vi "test SSL Client HTTPS Request to Google.vi"(8 "error in (no error)":errorcluster, 11 "TestCase in":refnum<class "test SSL Client.lvclass">) -> (0 "error out":errorcluster, 3 "TestCase out":refnum<class "test SSL Client.lvclass">)   [LabVIEW 2013, in "test SSL Client.lvclass"]
uses:
  test SSL Client.lvclass
  <vilib>/addons/_JKI Toolkits/VI Tester/TestCase.llb/TestCase.lvclass
  SSL_Lib/BIO/BIO.lvclass
  <vilib>/Wiresmith Technology/VITAC (VI Tester Advanced Comparisons)/VITAC.lvlib
  SSL_Lib/SSL-Context/SSL-Context.lvclass
  SSL_Lib/SSL/SSL.lvclass
  SSL_Lib/SSL/SSL_Mode.ctl
  suite SSL Client/suite SSL Client/SSL Context.vi
  suite SSL Client/suite SSL Client/suite SSL Client.lvclass
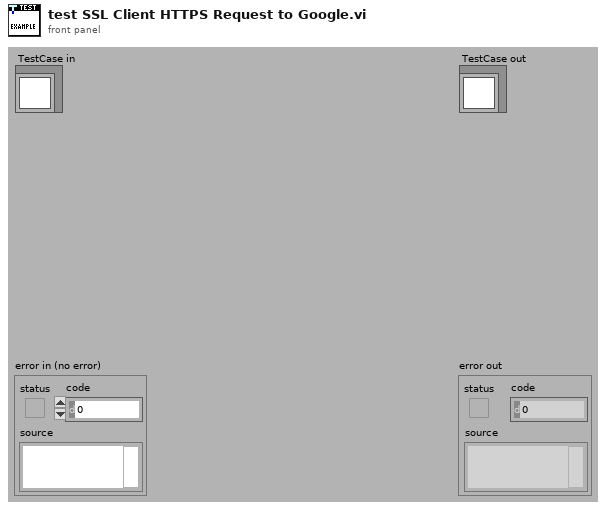
[diagram p1: front panel]
types:
  T1 = typedef "SSL_Lib.lvlib/SSL.lvclass/SSL_Mode.ctl" = i32
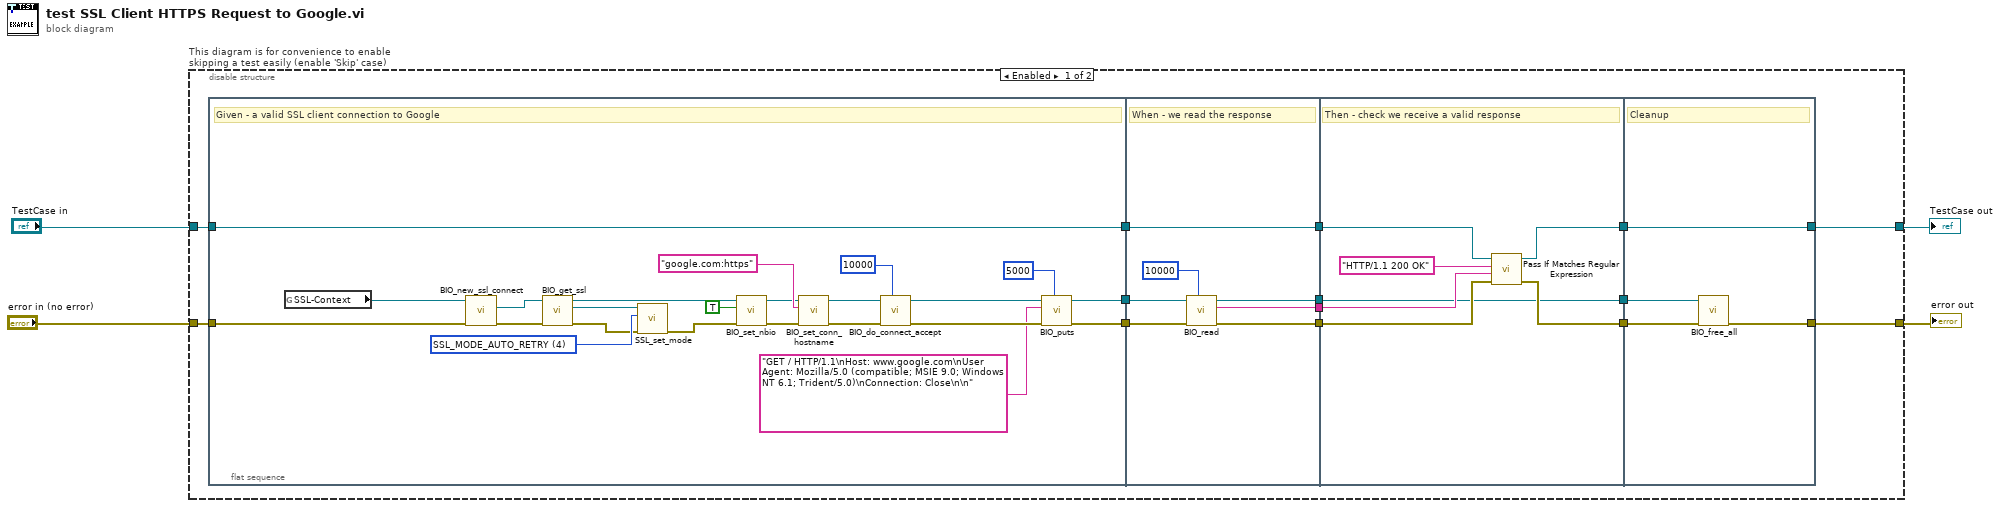
[diagram p0: block diagram]
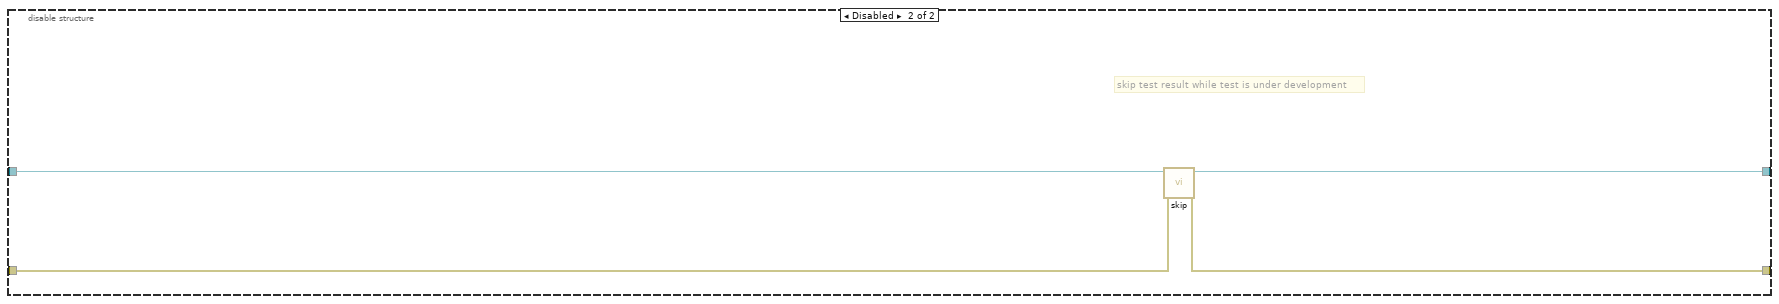
[diagram p2: hidden frame]
diagram:
  n1 = disable-structure "This diagram is for convenience to enable skipping a test easily (enable 'Skip' case)" shown="Enabled" {
    disable-tunnel: "TestCase in" -> [w12 w63]
    disable-tunnel: [w11 w61] -> w1
    disable-tunnel: [w10 w62] -> w3
    disable-tunnel: "error in (no error)" -> [w13 w60]
    frame Enabled {
      n2 = flat-sequence {
        tunnel: w13 -> [w27]
        tunnel: w12 -> [w36]
        tunnel: [w36] -> w18
        tunnel: [w35] -> w9
        tunnel: [w34] -> w8
        tunnel: [w48] -> w17
        tunnel: [w45] -> w16
        tunnel: w18 -> [w48]
        tunnel: w9 -> [w47]
        tunnel: w8 -> [w46]
        tunnel: [w44] -> w7
        tunnel: [w43] -> w6
        tunnel: [w53] -> w15
        tunnel: [w52] -> w14
        tunnel: w17 -> [w54]
        tunnel: w16 -> [w55]
        tunnel: w7 -> [w51]
        tunnel: w6 -> [w49]
        tunnel: [w49] -> w5
        tunnel: [w57] -> w10
        tunnel: [w59] -> w11
        tunnel: w15 -> [w59]
        tunnel: w14 -> [w58]
        tunnel: w5 -> [w56]
        frame #0 {
          w29 = T1 4 items=["None"=0, "SSL_MODE_ENABLE_PARTIAL_WRITE"=1, "SSL_MODE_ACCEPT_MOVING_WRITE_BUFFER"=2, "SSL_MODE_AUTO_RETRY"=4, "SSL_MODE_RELEASE_BUFFERS"=16, "SSL_MODE_SEND_FALLBACK_SCSV"=128] ("Mode")
          # "Given - a valid SSL client connection to Google"
          n3 = global read "SSL Context.vi" "SSL-Context"() -> (w26:refnum<class "SSL-Context.lvclass">)
          n4 = call "BIO_new_ssl_connect.vi"("error in (no error)"=w27, "SSL-Context in"=w26) -> ("error out"=w31:errorcluster, "BIO out"=w32:refnum<class "BIO.lvclass">)  [unwired: 7 in, 1 out]
          n5 = call "BIO_get_ssl.vi"("error in (no error)"=w31, "BIO in"=w32) -> ("error out"=w28:errorcluster, "SSL out"=w30:refnum<class "SSL.lvclass">, "BIO out"=w21:refnum<class "BIO.lvclass">)  [unwired: 7 in]
          n6 = call "SSL_set_mode.vi"("error in (no error)"=w28, "Mode"=w29, "SSL in"=w30) -> ("error out"=w24:errorcluster)  [unwired: 7 in, 1 out]
          n7 = call "BIO_set_nbio.vi"("error in (no error)"=w24, "Non-Blocking?"=TRUE, "BIO in"=w21) -> ("error out"=w22:errorcluster, "BIO out"=w23:refnum<class "BIO.lvclass">)  [unwired: 7 in]
          n8 = call "BIO_set_conn_hostname.vi"("error in (no error)"=w22, "Hostname"="google.com:https", "BIO in"=w23) -> ("error out"=w40:errorcluster, "BIO out"=w33:refnum<class "BIO.lvclass">)  [unwired: 7 in]
          n9 = call "BIO_do_connect_accept.vi"("Timeout (10000ms)"=u32 10000, "error in (no error)"=w40, "BIO in"=w33) -> ("error out"=w38:errorcluster, "BIO out"=w37:refnum<class "BIO.lvclass">)  [unwired: 7 in]
          n10 = call "BIO_puts.vi"("Timeout (10000ms)"=u32 5000, "error in (no error)"=w38, "String to write"="GET / HTTP/1.1\nHost: www.google.com\nUser Agent: Mozilla/5.0 (compatible; MSIE 9.0; Windows NT 6.1; Trident/5.0)\nConnection: Close\n\n", "BIO in"=w37) -> ("error out"=w35:errorcluster, "BIO out"=w34:refnum<class "BIO.lvclass">)  [unwired: 6 in]
        }
        frame #1 {
          # "When - we read the response"
          n11 = call "BIO_read.vi"("Timeout (10000ms)"=u32 10000, "error in (no error)"=w47, "BIO in"=w46) -> ("error out"=w45:errorcluster, "String read"=w44:string, "BIO out"=w43:refnum<class "BIO.lvclass">)  [unwired: 6 in]
        }
        frame #2 {
          # "Then - check we receive a valid response"
          n12 = call <vilib>:"Pass If Matches Regular Expression.vi"("error in (no error)"=w55, "actual"=w51, "regular expression"="HTTP/1.1 200 OK", "TestCase in"=w54) -> ("error out"=w52:errorcluster, "TestCase out"=w53:refnum<class "test SSL Client.lvclass">)  [unwired: 6 in]
        }
        frame #3 {
          # "Cleanup"
          n13 = call "BIO_free_all.vi"("error in (no error)"=w58, "BIO in"=w56) -> ("error out"=w57:errorcluster)  [unwired: 9 in]
        }
      }
    }
    frame Disabled {
      # "skip test result while test is under development"
      n14 = call <vilib>:"skip.vi"("error in (no error)"=w60, "TestCase in"=w63) -> ("error out"=w62:errorcluster, "TestCase out"=w61:refnum<class "test SSL Client.lvclass">)  [unwired: 8 in]
    }
  }
  "error out" <- w3
  "TestCase out" <- w1
